vi "Main Page.vi"(8 "error in (no error)":errorcluster, 11 "Node Ptr":T1 format="%.0x") -> (0 "error out":errorcluster)   [LabVIEW 2016, in "UDP Sender System Explorer.lvlib"]
uses:
  UDP Sender System Explorer.lvlib
  <vilib>/NI Veristand/Custom Device API/Custom Device Item Ref.ctl
  Shared/Constants.vi
  <vilib>/NI Veristand/Custom Device API/Get Item Property (U16).vi
  <vilib>/NI Veristand/Custom Device API/Get Item Property (String).vi
  <vilib>/NI Veristand/Custom Device API/Custom Device API.lvlib
  Shared/UDP Sender Shared.lvlib
panel:
  in  "Destination IP Address":string
  in  "Destination Port":u16
  out "UDP Channels Transmitted":i32(listbox)
  in  "Header":cluster{"Section Name":string}={"Section Name"="Custom Device Item Settings"}
  in  "Description":string
  in  "Name":string
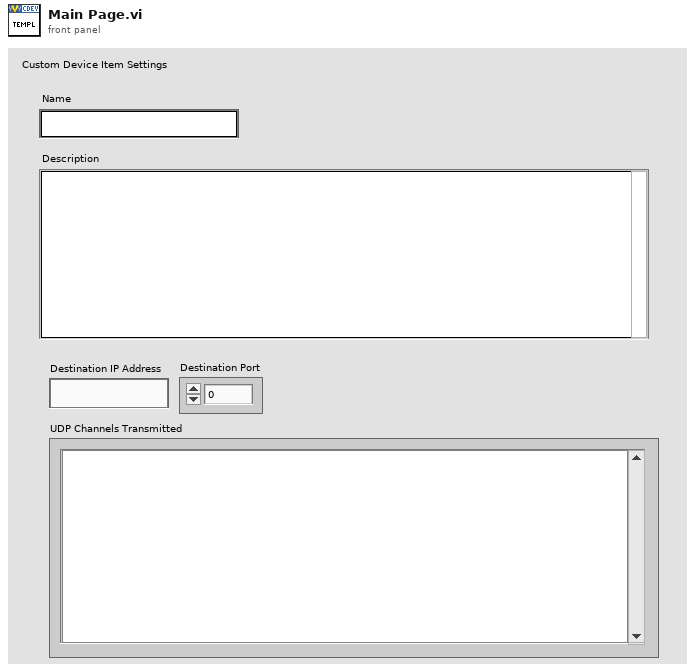
[diagram p1: front panel]
types:
  T1 = typedef "Custom Device API.lvlib/Custom Device Item Ref.ctl" = u64
  T2 = typedef "Custom Device API.lvlib/Custom Device Item Info.ctl" = cluster{"Name":string, "Is Channel":bool, "GUID":string, "Is Waveform":bool}
  T3 = typedef "Custom Device API.lvlib/Custom Device Commands.ctl" = enum16{"Default", "Item renamed", "Shutdown", "Dynamic button pressed"}
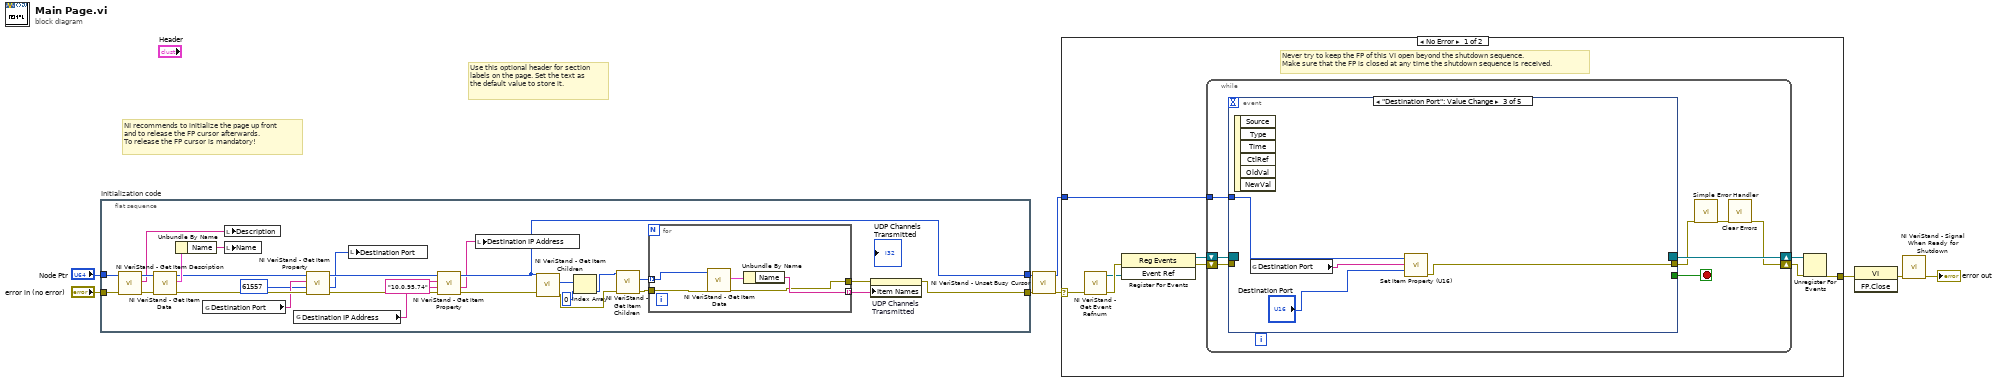
[diagram p0: block diagram]
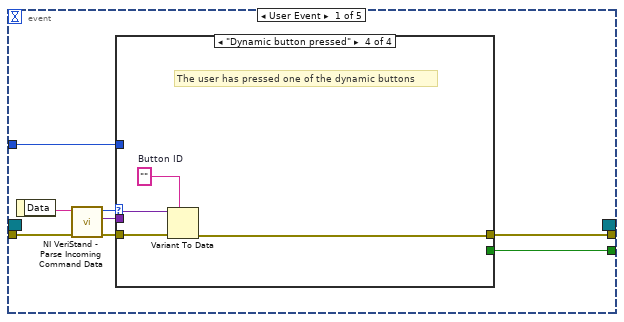
[diagram p2: hidden frame]
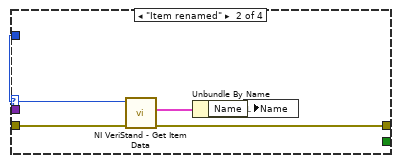
[diagram p4: hidden frame]
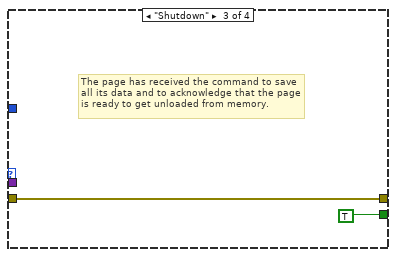
[diagram p5: hidden frame]
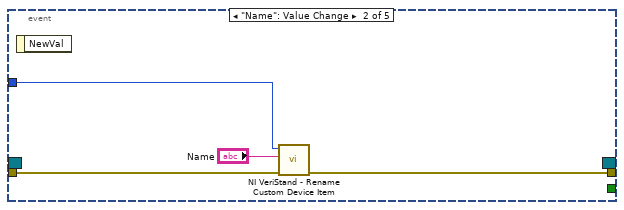
[diagram p6: hidden frame]
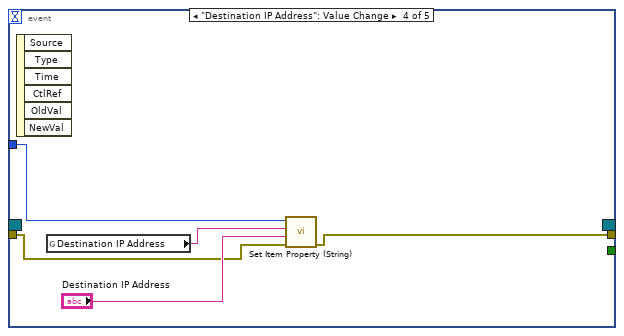
[diagram p7: hidden frame]
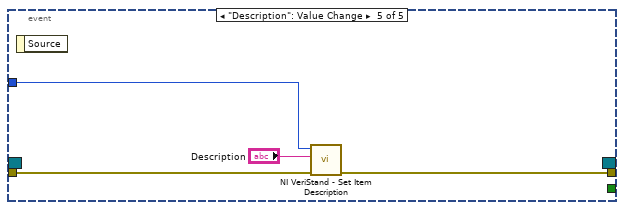
[diagram p8: hidden frame]
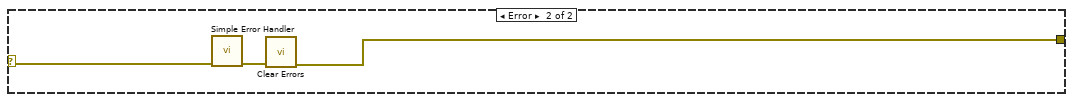
[diagram p9: hidden frame]
diagram:
  # "Use this optional header for section labels on the page. Set the text as the default value to store it."
  # "NI recommends to initialize the page up front\nand to release the FP cursor afterwards.\nTo release the FP cursor is mandatory!"
  n1 = flat-sequence "Initialization code" {
    tunnel: "error in (no error)" -> [w35]
    tunnel: "Node Ptr" -> [w34]
    tunnel: [w21] -> w4
    tunnel: [w15] -> w1
    frame #0 {
      n2 = call <vilib>:"NI VeriStand - Get Item Description.vi"("error in (no error)"=w35, "Item Ref in"=w34) -> ("error out"=w32:errorcluster, "Description"=w33:string, "Item Ref out"=w36:T1)  [unwired: 7 out]
      n3 = call <vilib>:"NI VeriStand - Get Item Data.vi"("error in (no error)"=w32, "Item Ref in"=w36) -> ("error out"=w20:errorcluster, "Item Info"=w31:T2, "Item Ref out"=w18:T1)  [unwired: 7 out]
      n4 = Unbundle By Name(w31) -> ("Name"=w30:string)
      n5 = global read "Constants.vi" "Destination Port"() -> (w14:string)
      n6 = local write "Description"(w33) -> ()
      n7 = local write "Name"(w30) -> ()
      n8 = global read "Constants.vi" "Destination IP Address"() -> (w10:string)
      n9 = call-poly <vilib>:"NI VeriStand - Get Item Property.vi"("error in (no error)"=w20, "Default Value"=u16 61557, "Property Name"=w14, "Item Ref in"=w18) -> ("error out"=w19:errorcluster, "Value"=w13:u16, "Item Ref out"=w16:T1)  [unwired: 4 in, 1 out]
      n10 = local write "Destination Port"(w13) -> ()
      n11 = call-poly <vilib>:"NI VeriStand - Get Item Property.vi"("error in (no error)"=w19, "Default Value"="10.0.95.74", "Property Name"=w10, "Item Ref in"=w16) -> ("error out"=w17:errorcluster, "Value"=w11:string, "Item Ref out"=w15:T1)  [unwired: 4 in, 1 out]
      n12 = local write "Destination IP Address"(w11) -> ()
      n13 = call <vilib>:"NI VeriStand - Get Item Children.vi"("error in (no error)"=w17, "Item Ref in"=w15) -> ("error out"=w26:errorcluster, "Child Refs"=w29:T1[])  [unwired: 6 in, 2 out]
      n14 = Index Array(array=w29, index=0) -> (element=w27:T1)
      n15 = call <vilib>:"NI VeriStand - Get Item Children.vi"("error in (no error)"=w26, "Item Ref in"=w27) -> ("error out"=w24:errorcluster, "Child Refs"=w25:T1[])  [unwired: 6 in, 2 out]
      n16 = for {
        tunnel: w25 -> [w41] mode=indexing
        tunnel: w24 -> [w40]
        tunnel: [w38] -> w23 mode=indexing
        tunnel: [w37] -> w22
        n17 = call <vilib>:"NI VeriStand - Get Item Data.vi"("error in (no error)"=w40, "Item Ref in"=w41) -> ("error out"=w37:errorcluster, "Item Info"=w39:T2)  [unwired: 6 in, 2 out]
        n18 = Unbundle By Name(w39) -> ("Name"=w38:string)
      }
      n19 = property on="UDP Channels Transmitted" class="LstBox (strict)"(error in=w22, "Item Names"=w23) -> (error out=w21:errorcluster)  [unwired: 1 in, 1 out]
    }
  }
  n20 = call <vilib>:"NI VeriStand - Unset Busy Cursor.vi"("error in (no error)"=w4) -> ("error out"=w3:errorcluster)  [unwired: 10 out]
  n21 = case shown="No Error" w3 {
    selector: w3 -> [w42 w98]
    tunnel: [w47 w96] -> w8
    tunnel: w1 -> [w43 _]
    frame No Error {
      # "Never try to keep the FP of this VI open beyond the shutdown sequence.\nMake sure that the FP is closed at any time the shutdown sequence is received."
      n22 = call <vilib>:"NI VeriStand - Get Event Refnum.vi"("error in (no error)"=w42) -> ("error out"=w50:errorcluster, "Event Ref"=w46:refnum<user-event>)  [unwired: 9 out]
      n23 = register-events(error in=w50, w46) -> (reference out=w44:refnum<event-registration>, error out=w45:errorcluster)  [unwired: 1 in]
      n24 = while {
        tunnel: w43 -> [w54]
        shift-right: [w51] -> w48
        shift-left: w45 -> [w57]
        shift-right: [w58] -> w49
        shift-left: w44 -> [w56]
        stop <- w55 stop-if-true
        n25 = event shown="[2] \"Destination Port\": Value Change" {
          selector: w56 -> [_ _ _ _ _]
          dyn-events: [_ _ _ _ _] -> w58
          timeout: _ -> [_ _ _ _ _]
          tunnel: w57 -> [w66 w82 _ w88 w94]
          tunnel: [w62 _ _ _ _] -> w55
          tunnel: [w61 w81 w83 w87 w93] -> w53
          tunnel: w54 -> [w60 w80 w86 w90 w95]
          event User Event {
            n26 = event-data() -> ("Data"=w65:string)  [unwired: 1 out]
            n27 = call <vilib>:"NI VeriStand - Parse Incoming Command Data.vi"("error in (no error)"=w66, "Incoming data"=w65) -> ("error out"=w64:errorcluster, "Outgoing data"=w59:variant, "Action"=w63:T3)  [unwired: 7 out]
            n28 = case shown="\"Dynamic button pressed\"" w63 {
              tunnel: w64 -> [w67 w72 w73 w78]
              tunnel: [_ _ TRUE _] -> w62
              tunnel: [w67 w69 w73 w75] -> w61
              tunnel: w60 -> [_ w71 _ _]
              tunnel: w59 -> [_ _ _ w77]
              frame "Default", Default {
              }
              frame "Item renamed" {
                n29 = call <vilib>:"NI VeriStand - Get Item Data.vi"("error in (no error)"=w72, "Item Ref in"=w71) -> ("error out"=w69:errorcluster, "Item Info"=w70:T2)  [unwired: 8 out]
                n30 = Unbundle By Name(w70) -> ("Name"=w68:string)
                n31 = local write "Name"(w68) -> ()
              }
              frame "Shutdown" {
                # "The page has received the command to save all its data and to acknowledge that the page is ready to get unloaded from memory."
              }
              frame "Dynamic button pressed" {
                w76 = ""  # Button ID
                # "The user has pressed one of the dynamic buttons"
                n32 = Variant To Data(error in=w78, type=w76, Variant=w77) -> (error out=w75:errorcluster)  [unwired: 1 out]
              }
            }
          }
          event "Name": Value Change {
            n33 = event-data() -> ()  [unwired: 2 out]
            n34 = call <vilib>:"NI VeriStand - Rename Custom Device Item.vi"("error in (no error)"=w82, "New Name"="Name", "Item Ref in"=w80) -> ("error out"=w81:errorcluster)  [unwired: 1 in, 7 out]
          }
          event "Destination Port": Value Change {
            n35 = event-data() -> ()  [unwired: 7 out]
            n36 = global read "Constants.vi" "Destination Port"() -> (w85:string)
            n37 = call <vilib>:"Set Item Property (U16).vi"("Value"="Destination Port", "Property Name"=w85, "Item Ref in"=w86) -> ("error out"=w83:errorcluster)  [unwired: 6 in, 2 out]
          }
          event "Destination IP Address": Value Change {
            n38 = event-data() -> ()  [unwired: 7 out]
            n39 = global read "Constants.vi" "Destination IP Address"() -> (w91:string)
            n40 = call <vilib>:"Set Item Property (String).vi"("error in (no error)"=w88, "Value"="Destination IP Address", "Property Name"=w91, "Item Ref in"=w90) -> ("error out"=w87:errorcluster)  [unwired: 5 in, 2 out]
          }
          event "Description": Value Change {
            n41 = event-data() -> ()  [unwired: 2 out]
            n42 = call <vilib>:"NI VeriStand - Set Item Description.vi"("error in (no error)"=w94, "Description"="Description", "Item Ref in"=w95) -> ("error out"=w93:errorcluster)  [unwired: 8 out]
          }
        }
        n43 = call <vilib>:"Simple Error Handler.vi"("error in (no error)"=w53) -> ("error out"=w52:errorcluster)  [unwired: 1 in, 7 out]
        n44 = call <vilib>:"Clear Errors.vi"("error in (no error)"=w52) -> ("error out"=w51:errorcluster)  [unwired: 1 in, 5 out]
      }
      n45 = Unregister For Events(event registration refnum=w49, error in=w48) -> (error out=w47:errorcluster)
    }
    frame Error {
      n46 = call <vilib>:"Simple Error Handler.vi"("error in (no error)"=w98) -> ("error out"=w97:errorcluster)  [unwired: 1 in, 7 out]
      n47 = call <vilib>:"Clear Errors.vi"("error in (no error)"=w97) -> ("error out"=w96:errorcluster)  [unwired: 1 in, 5 out]
    }
  }
  n48 = invoke class="VI" method="FP.Close"(error in=w8) -> (error out=w7:errorcluster)  [unwired: 2 in, 2 out]
  n49 = call <vilib>:"NI VeriStand - Signal When Ready for Shutdown.vi"("error in (no error)"=w7) -> ("error out"=→"error out":errorcluster)  [unwired: 10 out]
